vi "Close Device.vi"(8 "Error In":errorcluster, 11 "LINX Device Config":T1) -> (0 "Error Out":errorcluster, 3 "LINX Device Config":T1)   [LabVIEW 2020, in "Device.lvlib"]
doc: "Close the connection to the LINX device."
uses:
  Type Defs/LINX Device Config.ctl
  Type Defs/Interface.ctl
  Type Defs/TCP Config.ctl
  Type Defs/Channels.ctl
  Device.lvlib
  LMH-LINX.lvlib
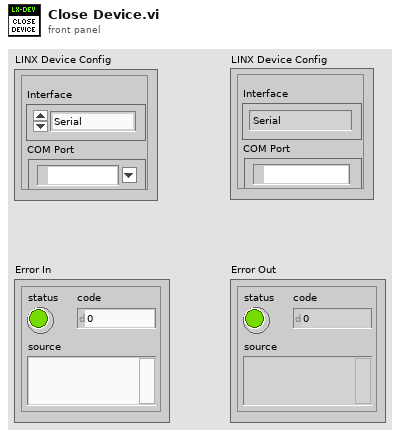
[diagram p1: front panel]
types:
  T1 = typedef "Device.lvlib/LINX Device Config.ctl" = cluster{"Interface":T2, "COM Port":refnum<visa-resource-name>, "TCP Configuration":T3, "Device Family":u8, "Device ID":u8, "Device Name":string, "TCP Ref":refnum<k5>, "Channels":T4}
  T2 = typedef "LMH-LINX.lvlib/Interface.ctl" = enum16{"Serial", "TCP"}
  T3 = typedef "Device.lvlib/TCP Config.ctl" = cluster{"IP Address":string, "Port":u16}
  T4 = typedef "LMH-LINX.lvlib/Channels.ctl" = cluster{"DI":u8[], "DO":u8[], "AI":u8[], "AO":u8[], "PWM":u8[], "QE":u8[], "UART":u8[], "I2C 2":u8[], "SPI":u8[], "CAN":u8[], "Servo":u8[], "AI Ref (V)":dbl, "AI Resolution (Bits)":u8, "AO Ref (V)":dbl, "AO Resolution (Bits)":u8}
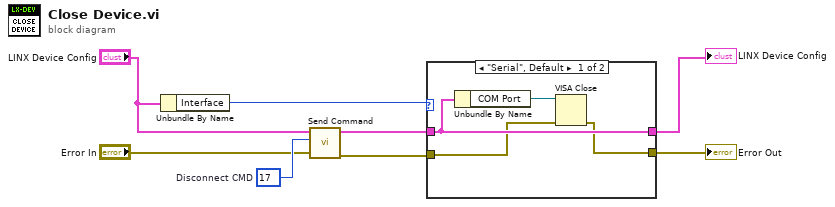
[diagram p0: block diagram]
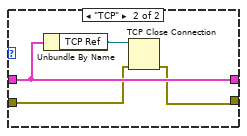
[diagram p2: hidden frame]
diagram:
  w5 = u16 17  # Disconnect CMD
  n1 = Unbundle By Name("LINX Device Config") -> ("Interface"=w7:T2)
  n2 = call "Send Command.vi"("Error In"="Error In", "CMD"=w5, "LINX Device Config"="LINX Device Config") -> ("Error Out"=w1:errorcluster, "LINX Device Config"=w3:T1)  [unwired: 5 in, 2 out]
  n3 = case shown="\"Serial\", Default" w7 {
    tunnel: w3 -> [w11 w16]
    tunnel: w1 -> [w10 w13]
    tunnel: [w9 w14] -> w8
    tunnel: [w11 w16] -> w6
    frame "Serial", Default {
      n4 = Unbundle By Name(w11) -> ("COM Port"=w12:refnum<visa-resource-name>)
      n5 = VISA Close(VISA resource name=w12, error in (no error)=w10) -> (error out=w9:errorcluster)
    }
    frame "TCP" {
      n6 = Unbundle By Name(w16) -> ("TCP Ref"=w15:refnum<k5>)
      n7 = TCP Close Connection(connection ID=w15, error in (no error)=w13) -> (error out=w14:errorcluster)  [unwired: 1 in, 1 out]
    }
  }
  "Error Out" <- w8
  "LINX Device Config" <- w6
